vi "Read Oxygen Oil Presence.vi"(0 "Session Handle in":T1, 11 "error in (no error)":errorcluster) -> (4 "Session Handle out":T1, 6 "Present?":bool, 15 "error out":errorcluster)   [LabVIEW 2015, in "Gas.lvclass"]
uses:
  Gas.lvclass
  Typedefs/Session Handle.ctl
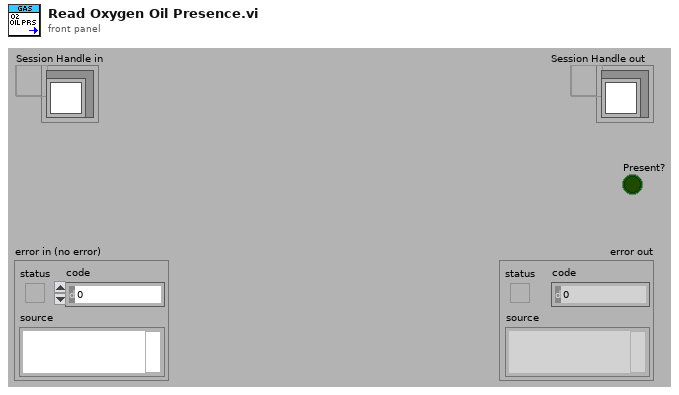
[diagram p1: front panel]
types:
  T1 = typedef "Gas.lvclass/Session Handle.ctl" = refnum<data-value>
  T2 = typedef "XNET Frame CAN.ctl" = cluster{"timestamp":timestamp, "payload":u8[], "identifier":u32, "type":T3, "extended?":bool, "echo?":bool}
  T3 = typedef "XNET Frame Type CAN.ctl" = u8
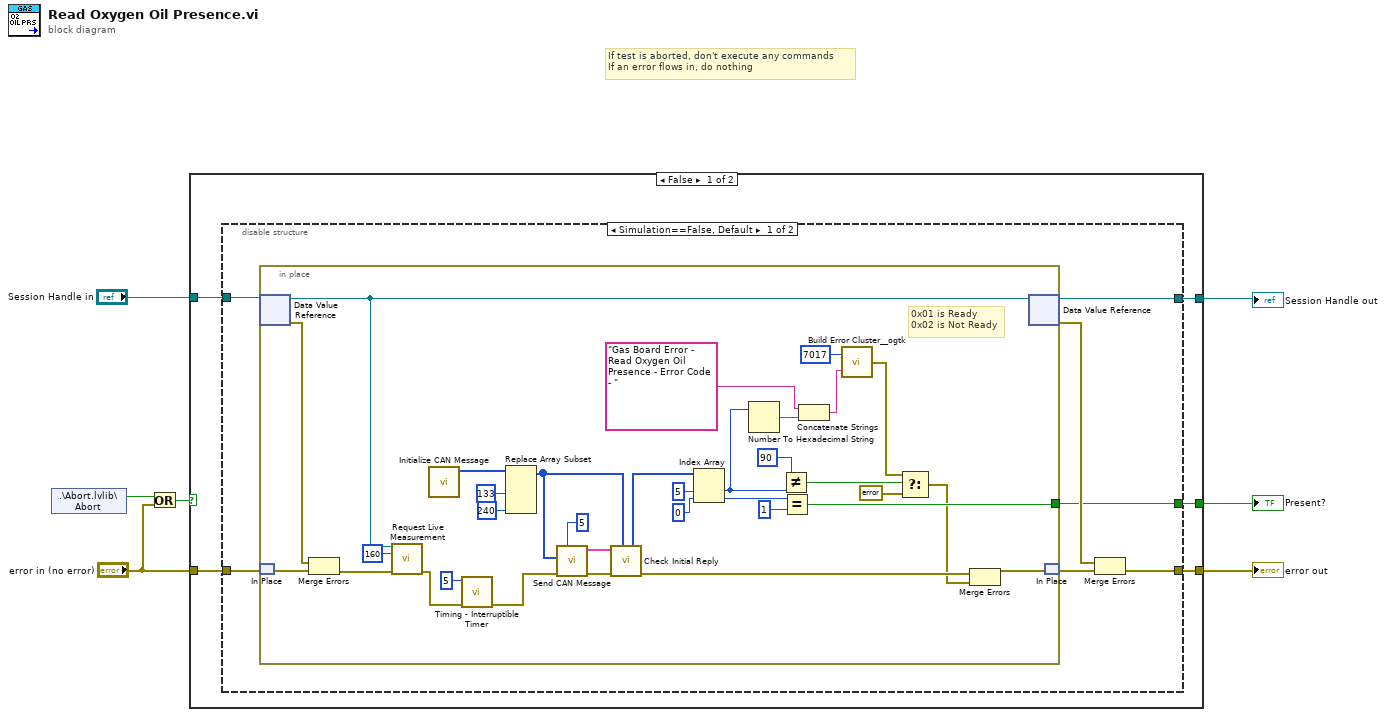
[diagram p0: block diagram]
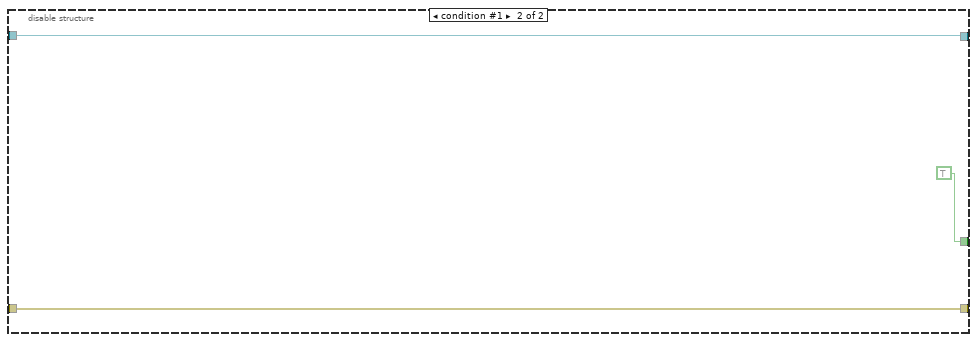
[diagram p2: hidden frame]
diagram:
  # "If test is aborted, don't execute any commands\nIf an error flows in, do nothing"
  n1 = shared-variable ".\\Abort.lvlib\\Abort"() -> (w4:bool)  [unwired: 1 in, 1 out]
  n2 = Or(x=w4, y="error in (no error)") -> (x .or. y?=w2:bool)
  n3 = case shown="False" w2 {
    tunnel: [w12 w57] -> w6
    tunnel: [w11 w56] -> w5
    tunnel: "Session Handle in" -> [w10 w57]
    tunnel: "error in (no error)" -> [w9 w56]
    tunnel: [w8 _] -> w1
    frame False {
      n4 = disable-structure shown="Simulation==False, Default" {
        disable-tunnel: [w19 w55] -> w12
        disable-tunnel: [w16 w54] -> w11
        disable-tunnel: w10 -> [w15 w55]
        disable-tunnel: w9 -> [w14 w54]
        disable-tunnel: [w13 TRUE] -> w8
        frame condition #0 (active) {
          n5 = in-place {
            in-place-border: [w34] -> w13
            # "0x01 is Ready\n0x02 is Not Ready"
            n6 = in-place-dvr #1(w15) -> (w27:refnum<class "Gas.lvclass">, w47:errorcluster)
            n7 = in-place-match #2(w14) -> (w46:errorcluster)
            n8 = Merge Errors(w47, w46) -> (w28:errorcluster)
            n9 = call "Request Live Measurement.vi"("Gas In"=w27, "Request Type"=u8 160, "error in (no error)"=w28) -> ("error out"=w25:errorcluster)  [unwired: 10 in, 2 out]
            n10 = call "Initialize CAN Message.vi"() -> ("Initial Payload"=w49:u8[])  [unwired: 11 in]
            n11 = call "Timing - Interruptible Timer.vi"("error in (no error)"=w25, "Wait (s)"=5) -> ("error out"=w23:errorcluster)  [unwired: 7 in, 2 out]
            n12 = Replace Array Subset(array=w49, new element #1=u8 133 ("new element/subarray"), new element #2=u8 240 ("new element/subarray")) -> (w45:u8[])  [unwired: 2 in]
            n13 = call "Send CAN Message.vi"("Number of Retries"=5, "error in (no error)"=w23, "payload"=w45) -> ("error out"=w22:errorcluster, "Reply"=w43:T2[])  [unwired: 6 in, 1 out]
            n14 = call "Check Initial Reply.vi"("Write Message"=w45, "error in (no error)"=w22, "Reply"=w43) -> ("error out"=w21:errorcluster, "Data Packet"=w48:u8[])  [unwired: 5 in, 2 out]
            n15 = Index Array(array=w48, index #1=5 ("index"), index #2=0 ("index")) -> (element #1=w33:u8, element #2=w36:u8)
            n16 = Number To Hexadecimal String(2:w33) -> (0:w31:string)  [unwired: 1 in]
            n17 = Not Equal?(x=u8 90 ("new element/subarray"), y=w33) -> (x != y?=w39:bool)
            n18 = Equal?(x=w36, y=u8 1) -> (x = y?=w34:bool)
            n19 = Concatenate Strings("Gas Board Error - Read Oxygen Oil Presence - Error Code - " ("string"), w31) -> (w29:string)
            n20 = call <userlib>:"Build Error Cluster__ogtk.vi"("String to Prepend to source (\"\")"=w29, "code"=7017) -> ("error out"=w41:errorcluster)
            n21 = Select(t=w41, s=w39, f=errorcluster {"status"=FALSE, "code"=0, "source"=""}) -> (s? t:f=w20:errorcluster)
            n22 = Merge Errors(w21, w20) -> (w50:errorcluster)
            n23 = in-place-dvr #1(w27) -> (w19:T1, w17:errorcluster)
            n24 = in-place-match #2(w50) -> (w18:errorcluster)
          }
          n25 = Merge Errors(w17, w18) -> (w16:errorcluster)
        }
        frame condition #1 {
        }
      }
    }
    frame True {
    }
  }
  "Session Handle out" <- w6
  "error out" <- w5
  "Present?" <- w1
